vi "Select Library by Pathname.vi"(8 "error in":errorcluster, 10 "Path to Library":path, 11 "All Libraries In":refnum<vi>[](array[refnum])) -> (0 "error out":errorcluster, 2 "Selected Library":refnum<vi>, 3 "All Libraries Out":refnum<vi>[](array[refnum]))   [LabVIEW 2017, in "Shared Variables Library.lvlib"]
doc: "Selects a single library, from an array of library references.\n\nThe given path is used to select the desired reference."
uses:
  Shared Variables Library.lvlib
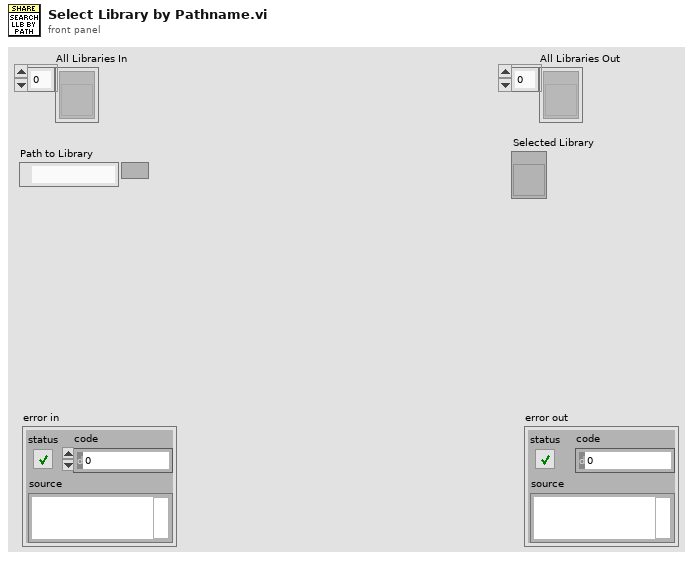
[diagram p1: front panel]
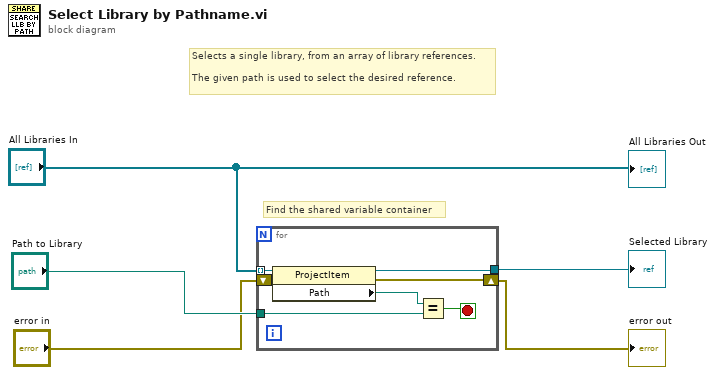
[diagram p0: block diagram]
diagram:
  # "Selects a single library, from an array of library references.\n\nThe given path is used to select the desired reference."
  # "Find the shared variable container"
  n1 = for {
    tunnel: "All Libraries In" -> [w12] mode=indexing
    tunnel: [w9] -> w1
    shift-right: [w8] -> w2
    shift-left: "error in" -> [w7]
    tunnel: "Path to Library" -> [w6]
    stop <- w10 stop-if-true
    n2 = property class="ProjectItem"(reference=w12, error in=w7) -> (reference out=w9:refnum<vi>, error out=w8:errorcluster, "Path"=w11:path)
    n3 = Equal?(x=w11, y=w6) -> (x = y?=w10:bool)
  }
  "error out" <- w2
  "Selected Library" <- w1
  "All Libraries Out" <- "All Libraries In"
